vi "LinearSystemId_CreateFlywheelSystem.vi"(9 "G":dbl, 10 "jKgMetersSquared":dbl, 11 "DCMOTOR":T1 {"Kt_NMPerAmp" format="%13.5p"; "Kv_RadPerSecPerVolt" format="%13.5p"; "R_Ohms" format="%13.5p"; "FreeSpeed_RadPerSec" format="%13.5p"; "FreeCurrent_Amps" format="%13.5p"; "StallCurrent_Amps" format="%13.5p"; "StallTorque_NM" format="%13.5p"; "nominalVoltage_Volts" format="%13.5p"}) -> (3 "Linearsystem":T2)   [LabVIEW 2019, in "Trajectory_Library.lvlib"]
doc: "Creates a new LINEAR SYSTEM data cluster with the specified values. \n\n\nInputs: \n - XXX -- XXX.\n\nOutputs:\n - XXX -- XXX."
uses:
  Trajectory_Library.lvlib
  LINEAR_SYSTEM.ctl
  <vilib>/Analysis/Matrix/Datatypes/RealMatrix.ctl
  DCMOTOR.CTL
  <vilib>/Analysis/7linalg.llb/Create Special Real Matrix.vi
  <vilib>/Analysis/NI_AALPro.lvlib
  <vilib>/Analysis/Matrix/NI_Matrix.lvlib
panel:
  in  "Outputs":i32=1
  in  "Inputs":i32=1
  in  "States":i32=1
  # "<States,States>"
  # "<States,Inputs>"
  # "<Outputs,States>"
  # "<Outputs,Inputs>"
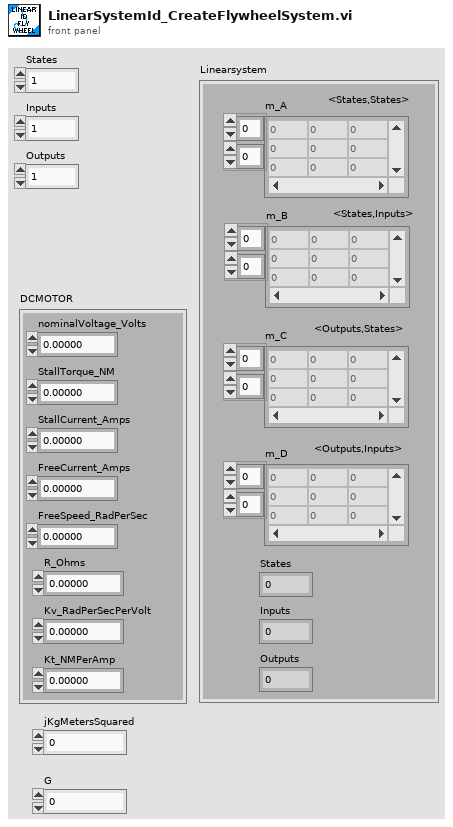
[diagram p1: front panel]
types:
  T1 = typedef "Trajectory_Library.lvlib/DCMOTOR.CTL" = cluster{"nominalVoltage_Volts":dbl, "StallTorque_NM":dbl, "StallCurrent_Amps":dbl, "FreeCurrent_Amps":dbl, "FreeSpeed_RadPerSec":dbl, "R_Ohms":dbl, "Kv_RadPerSecPerVolt":dbl, "Kt_NMPerAmp":dbl}
  T2 = typedef "Trajectory_Library.lvlib/LINEAR_SYSTEM.ctl" = cluster{"m_A":T3, "m_B":T3, "m_C":T3, "m_D":T3, "States":i32, "Inputs":i32, "Outputs":i32}
  T3 = typedef "NI_Matrix.lvlib/RealMatrix.ctl" = dbl[][]
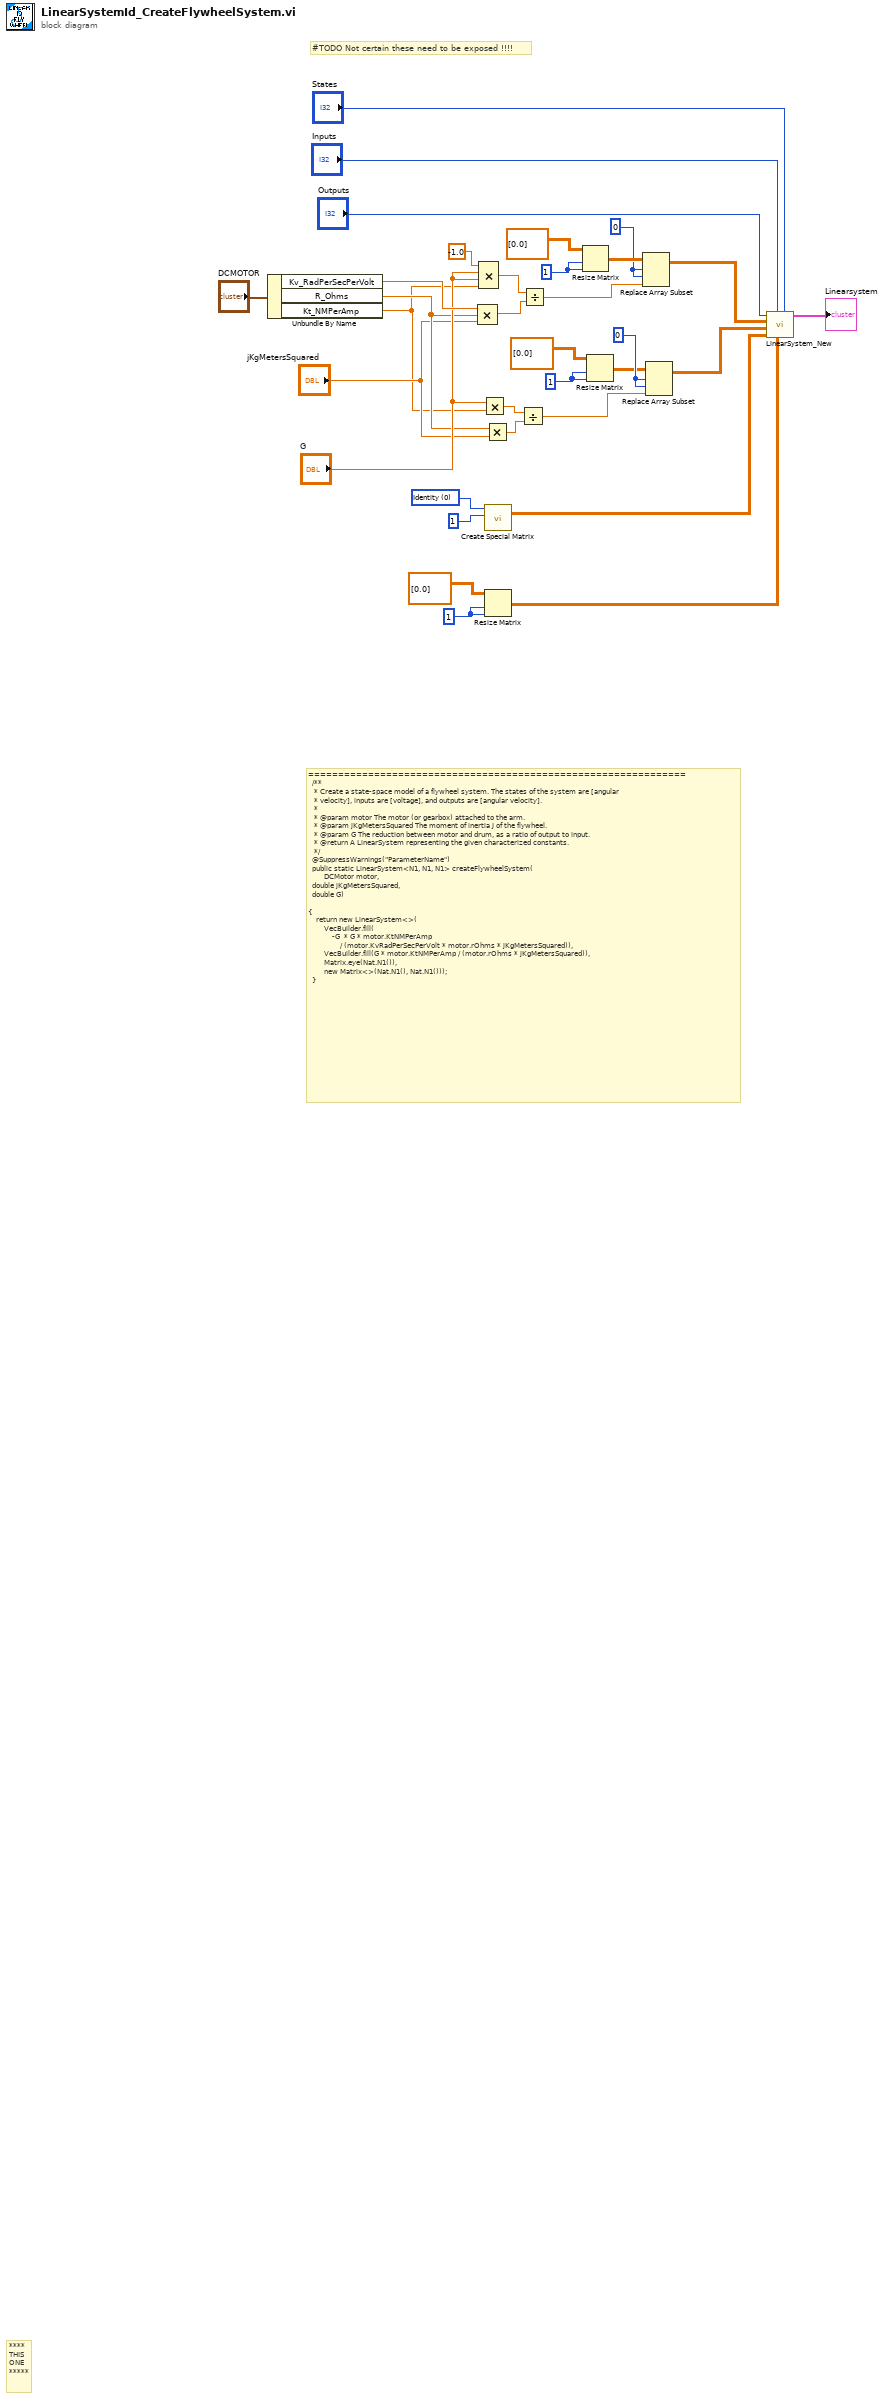
[diagram p0: block diagram]
diagram:
  w11 = 0 ("index (col)")
  w13 = 0 ("index (col)")
  w18 = 1 ("number of rows")
  w20 = 1 ("number of rows")
  w24 = 1 ("number of rows")
  w26 = 0 items=["Identity", "Diagonal", "Toeplitz", "Vandermonde", "Companion", "Hankel", "Hadamard", "Wilkinson", "Hilbert", "Inverse Hilbert", "Rosser", "Pascal"] ("matrix type")
  # "#TODO Not certain these need to be exposed !!!!"
  # "===============================================================\n  /**\n   * Create a state-space model of a flywheel system. The states of the system are [angular\n   * velocity], inputs are [voltage], and outputs are [angular velocity].\n   *\n   * @param motor The motor (or gearbox) attached to the arm.\n   * @param jKgMetersSquared The moment of inertia J of the flywheel.\n   * @param G The reduction between motor and drum, as a ratio of output to input.\n   * @return A LinearSystem representing the given characterized constants.\n   */\n  @SuppressWarnings(\"ParameterName\")\n  public static LinearSystem<N1, N1, N1> createFlywheelSystem(\n      \t\tDCMotor motor, \n\t\tdouble jKgMetersSquared, \n\t\tdouble G) \n\n{\n    return new LinearSystem<>(\n        VecBuilder.fill(\n            -G  * G * motor.KtNMPerAmp\n                / (motor.KvRadPerSecPerVolt * motor.rOhms * jKgMetersSquared)),\n        VecBuilder.fill(G * motor.KtNMPerAmp / (motor.rOhms * jKgMetersSquared)),\n        Matrix.eye(Nat.N1()),\n        new Matrix<>(Nat.N1(), Nat.N1()));\n  }"
  # "****\nTHIS\nONE\n*****"
  n1 = Unbundle By Name("DCMOTOR") -> ("Kv_RadPerSecPerVolt"=w27:dbl, "R_Ohms"=w8:dbl, "Kt_NMPerAmp"=w1:dbl)
  n2 = Compound Arithmetic op=MULTIPLY(w27, w8, "jKgMetersSquared") -> (w15:dbl)
  n3 = Compound Arithmetic op=MULTIPLY(-1.0 ("value"), "G", "G", w1) -> (w16:dbl)
  n4 = Multiply(x="G", y=w1) -> (x*y=w6:dbl)
  n5 = Multiply(x=w8, y="jKgMetersSquared") -> (x*y=w5:dbl)
  n6 = call-poly <vilib>:"Create Special Matrix.vi"("matrix type"=w26, "matrix size"=1) -> ("Special Matrix"=w21:T3)  [unwired: 3 in, 1 out]
  n7 = Resize Matrix(1:w24, 2:w24, 4:T3 [[0.0]] ("matrix")) -> (0:w22:T3)
  n8 = Divide(x=w6, y=w5) -> (x/y=w4:dbl)
  n9 = Divide(x=w16, y=w15) -> (x/y=w12:dbl)
  n10 = Resize Matrix(1:w20, 2:w20, 4:T3 [[0.0]] ("matrix")) -> (0:w14:T3)
  n11 = Resize Matrix(1:w18, 2:w18, 4:T3 [[0.0]] ("matrix")) -> (0:w10:T3)
  n12 = Replace Array Subset(array=w14, new element=w12, index (row)=w13, index (col)=w13) -> (w3:T3)
  n13 = Replace Array Subset(array=w10, new element=w4, index (row)=w11, index (col)=w11) -> (w2:T3)
  n14 = call "LinearSystem_New.vi"("States"="States", "D"=w22, "Inputs"="Inputs", "C"=w21, "B"=w2, "A"=w3, "Outputs"="Outputs") -> ("Linearsystem"=→"Linearsystem":T2)  [unwired: 4 in]
